vi "故障告警分析.vi"(8 "告警代码":u16, 9 "故障代码":u16, 10 "运行步序":u16, 11 "参数":string) -> (2 "报警内容":T1, 3 "简易报警状态":cluster{"故障状态":string, "报警状态":string})   [LabVIEW 2016, in "斯坦道总氮.lvlib"]
panel:
  # "1、注射泵水样阀口堵塞；\n2、注射泵阀过载或丝杆无动作。"
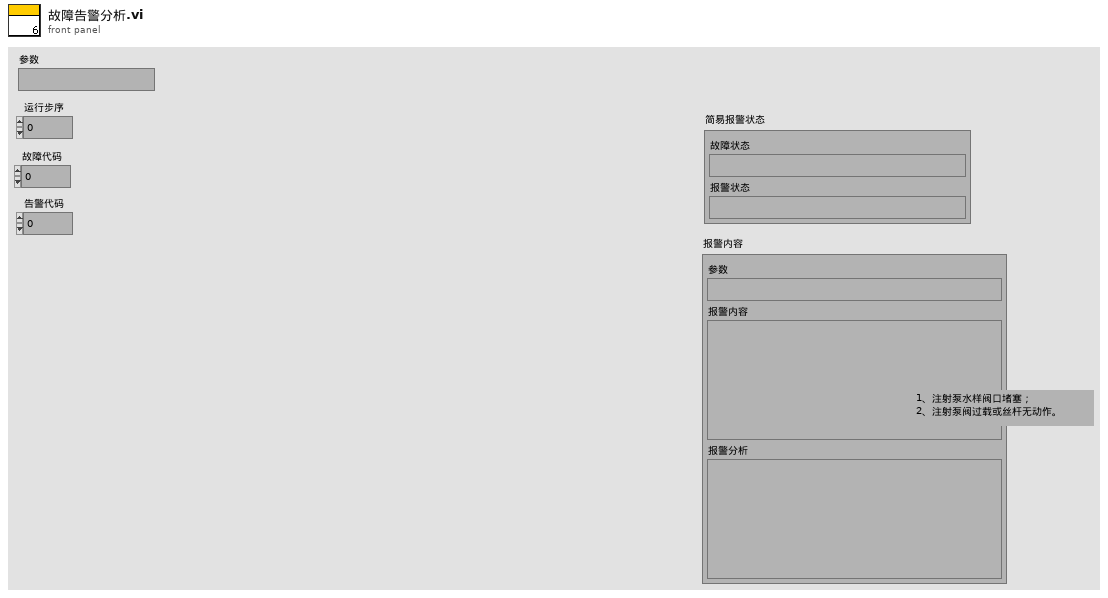
[diagram p1: front panel]
types:
  T1 = cluster{"参数":string, "报警内容":string, "报警分析":string}
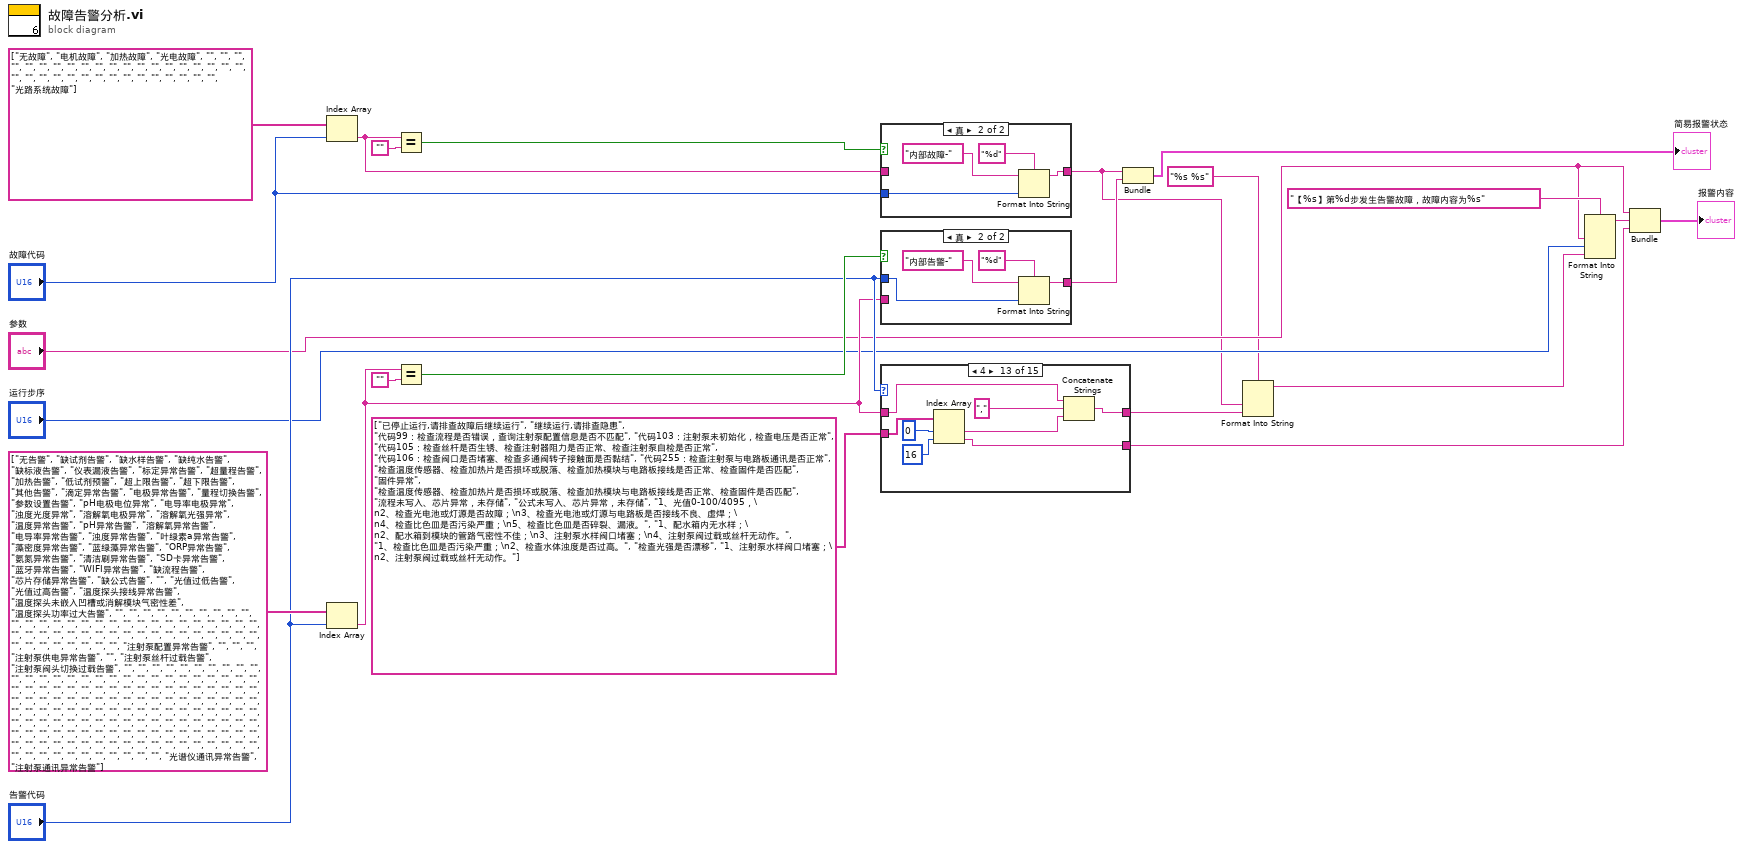
[diagram p0: block diagram]
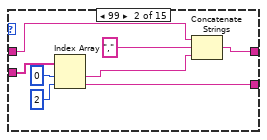
[diagram p3: hidden frame]
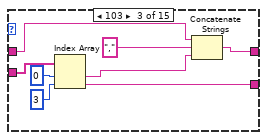
[diagram p4: hidden frame]
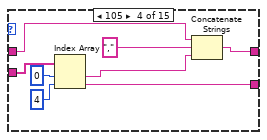
[diagram p5: hidden frame]
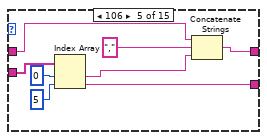
[diagram p6: hidden frame]
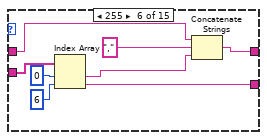
[diagram p7: hidden frame]
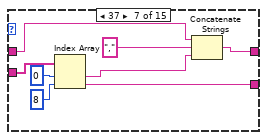
[diagram p8: hidden frame]
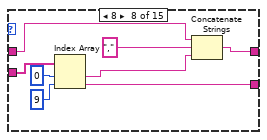
[diagram p9: hidden frame]
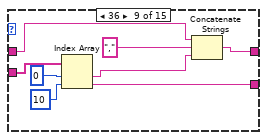
[diagram p10: hidden frame]
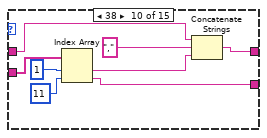
[diagram p11: hidden frame]
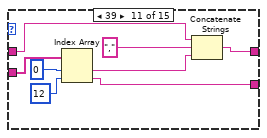
[diagram p12: hidden frame]
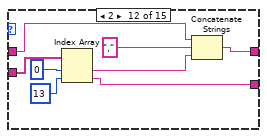
[diagram p13: hidden frame]
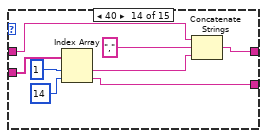
[diagram p14: hidden frame]
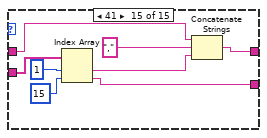
[diagram p15: hidden frame]
diagram:
  n1 = Index Array(array=string[] ["无故障", "电机故障", "加热故障", "光电故障", "", "", "", "", "", "", "", "", "", "", "", "", "", "", "", "", "", "", "", "", "", "", "", "", "", "", "", "", "", "", "", "", "", "", "", "光路系统故障"], index="故障代码") -> (element=w20:string)
  n2 = Index Array(array=string[] ["无告警", "缺试剂告警", "缺水样告警", "缺纯水告警", "缺标液告警", "仪表漏液告警", "标定异常告警", "超量程告警", "加热告警", "低试剂预警", "超上限告警", "超下限告警", "其他告警", "滴定异常告警", "电极异常告警", "量程切换告警", "参数设置告警", "pH电极电位异常", "电导率电极异常", "浊度光度异常", "溶解氧电极异常", "溶解氧光强异常", "温度异常告警", "pH异常告警", "溶解氧异常告警", "电导率异常告警", "浊度异常告警", "叶绿素a异常告警", "藻密度异常告警", "蓝绿藻异常告警", "ORP异常告警", "氨氮异常告警", "清洁刷异常告警", "SD卡异常告警", "蓝牙异常告警", "WIFI异常告警", "缺流程告警", "芯片存储异常告警", "缺公式告警", "", "光值过低告警", "光值过高告警", "温度探头接线异常告警", "温度探头未嵌入凹槽或消解模块气密性差", "温度探头功率过大告警", "", "", "", "", "", "", "", "", "", "", "", "", "", "", "", "", "", "", "", "", "", "", "", "", "", "", "", "", "", "", "", "", "", "", "", "", "", "", "", "", "", "", "", "", "", "", "", "", "", "", "", "", "", "", "注射泵配置异常告警", "", "", "", "注射泵供电异常告警", "", "注射泵丝杆过载告警", "注射泵阀头切换过载告警", "", "", "", "", "", "", "", "", "", "", "", "", "", "", "", "", "", "", "", "", "", "", "", "", "", "", "", "", "", "", "", "", "", "", "", "", "", "", "", "", "", "", "", "", "", "", "", "", "", "", "", "", "", "", "", "", "", "", "", "", "", "", "", "", "", "", "", "", "", "", "", "", "", "", "", "", "", "", "", "", "", "", "", "", "", "", "", "", "", "", "", "", "", "", "", "", "", "", "", "", "", "", "", "", "", "", "", "", "", "", "", "", "", "", "", "", "", "", "", "", "", "", "", "", "", "", "", "", "", "", "", "", "", "", "", "", "", "", "", "", "", "", "", "", "", "", "", "光谱仪通讯异常告警", "注射泵通讯异常告警"], index="告警代码") -> (element=w13:string)
  n3 = Equal?(x=w20, y="") -> (x = y?=w21:bool)
  n4 = Equal?(x=w13, y="") -> (x = y?=w16:bool)
  n5 = case shown="真" w21 {
    tunnel: [w24 w26] -> w2
    tunnel: w20 -> [w24 _]
    tunnel: "故障代码" -> [_ w25]
    frame False {
    }
    frame True {
      n6 = Format Into String(format string="%d" ("格式字符串"), initial string="内部故障-" ("工作状态"), w25) -> (resulting string=w26:string)  [unwired: 1 in, 1 out]
    }
  }
  n7 = case shown="真" w16 {
    tunnel: [w29 w31] -> w12
    tunnel: w13 -> [w29 _]
    tunnel: "告警代码" -> [_ w30]
    frame False {
    }
    frame True {
      n8 = Format Into String(format string="%d" ("格式字符串"), initial string="内部告警-" ("工作状态"), w30) -> (resulting string=w31:string)  [unwired: 1 in, 1 out]
    }
  }
  n9 = case shown="4" "告警代码" {
    tunnel: string[] ["已停止运行,请排查故障后继续运行", "继续运行,请排查隐患", "代码99：检查流程是否错误，查询注射泵配置信息是否不匹配", "代码103：注射泵未初始化，检查电压是否正常", "代码105：检查丝杆是否生锈、检查注射器阻力是否正常、检查注射泵自检是否正常", "代码106：检查阀口是否堵塞、检查多通阀转子接触面是否黏结", "代码255：检查注射泵与电路板通讯是否正常", "检查温度传感器、检查加热片是否损坏或脱落、检查加热模块与电路板接线是否正常、检查固件是否匹配", "固件异常", "检查温度传感器、检查加热片是否损坏或脱落、检查加热模块与电路板接线是否正常、检查固件是否匹配", "流程未写入、芯片异常，未存储", "公式未写入、芯片异常，未存储", "1、光值0-100/4095，\n2、检查光电池或灯源是否故障；\n3、检查光电池或灯源与电路板是否接线不良、虚焊；\n4、检查比色皿是否污染严重；\n5、检查比色皿是否碎裂、漏液。", "1、配水箱内无水样；\n2、配水箱到模块的管路气密性不佳；\n3、注射泵水样阀口堵塞；\n4、注射泵阀过载或丝杆无动作。", "1、检查比色皿是否污染严重；\n2、检查水体浊度是否过高。", "检查光强是否漂移", "1、注射泵水样阀口堵塞；\n2、注射泵阀过载或丝杆无动作。"] -> [_ w42 w50 w58 w66 w74 w82 w90 w98 w106 w114 w122 w130 w138 w146]
    tunnel: [w34 w37 w45 w53 w61 w69 w77 w85 w93 w101 w109 w117 w125 w133 w141] -> w3
    tunnel: [_ w38 w46 w54 w62 w70 w78 w86 w94 w102 w110 w118 w126 w134 w142] -> w10
    tunnel: w13 -> [w34 w36 w44 w52 w60 w68 w76 w84 w92 w100 w108 w116 w124 w132 w140]
    frame 0, Default {
    }
    frame 99 {
      n10 = Index Array(array=w42, index #1=0 ("索引"), index #2=2 ("索引")) -> (element #1=w40:string, element #2=w38:string)
      n11 = Concatenate Strings(w36, "," ("字符串"), w40) -> (w37:string)
    }
    frame 103 {
      n12 = Index Array(array=w50, index #1=0 ("索引"), index #2=3 ("索引")) -> (element #1=w48:string, element #2=w46:string)
      n13 = Concatenate Strings(w44, "," ("字符串"), w48) -> (w45:string)
    }
    frame 105 {
      n14 = Index Array(array=w58, index #1=0 ("索引"), index #2=4 ("索引")) -> (element #1=w56:string, element #2=w54:string)
      n15 = Concatenate Strings(w52, "," ("字符串"), w56) -> (w53:string)
    }
    frame 106 {
      n16 = Index Array(array=w66, index #1=0 ("索引"), index #2=5 ("索引")) -> (element #1=w64:string, element #2=w62:string)
      n17 = Concatenate Strings(w60, "," ("字符串"), w64) -> (w61:string)
    }
    frame 255 {
      n18 = Index Array(array=w74, index #1=0 ("索引"), index #2=6 ("索引")) -> (element #1=w72:string, element #2=w70:string)
      n19 = Concatenate Strings(w68, "," ("字符串"), w72) -> (w69:string)
    }
    frame 37 {
      n20 = Index Array(array=w82, index #1=0 ("索引"), index #2=8 ("索引")) -> (element #1=w80:string, element #2=w78:string)
      n21 = Concatenate Strings(w76, "," ("字符串"), w80) -> (w77:string)
    }
    frame 8 {
      n22 = Index Array(array=w90, index #1=0 ("索引"), index #2=9 ("索引")) -> (element #1=w88:string, element #2=w86:string)
      n23 = Concatenate Strings(w84, "," ("字符串"), w88) -> (w85:string)
    }
    frame 36 {
      n24 = Index Array(array=w98, index #1=0 ("索引"), index #2=10 ("索引")) -> (element #1=w96:string, element #2=w94:string)
      n25 = Concatenate Strings(w92, "," ("字符串"), w96) -> (w93:string)
    }
    frame 38 {
      n26 = Index Array(array=w106, index #1=1 ("索引"), index #2=11 ("索引")) -> (element #1=w104:string, element #2=w102:string)
      n27 = Concatenate Strings(w100, "," ("字符串"), w104) -> (w101:string)
    }
    frame 39 {
      n28 = Index Array(array=w114, index #1=0 ("索引"), index #2=12 ("索引")) -> (element #1=w112:string, element #2=w110:string)
      n29 = Concatenate Strings(w108, "," ("字符串"), w112) -> (w109:string)
    }
    frame 2 {
      n30 = Index Array(array=w122, index #1=0 ("索引"), index #2=13 ("索引")) -> (element #1=w120:string, element #2=w118:string)
      n31 = Concatenate Strings(w116, "," ("字符串"), w120) -> (w117:string)
    }
    frame 4 {
      n32 = Index Array(array=w130, index #1=0 ("索引"), index #2=16 ("索引")) -> (element #1=w128:string, element #2=w126:string)
      n33 = Concatenate Strings(w124, "," ("字符串"), w128) -> (w125:string)
    }
    frame 40 {
      n34 = Index Array(array=w138, index #1=1 ("索引"), index #2=14 ("索引")) -> (element #1=w136:string, element #2=w134:string)
      n35 = Concatenate Strings(w132, "," ("字符串"), w136) -> (w133:string)
    }
    frame 41 {
      n36 = Index Array(array=w146, index #1=1 ("索引"), index #2=15 ("索引")) -> (element #1=w144:string, element #2=w142:string)
      n37 = Concatenate Strings(w140, "," ("字符串"), w144) -> (w141:string)
    }
  }
  n38 = Bundle(w2, w12) -> (→"简易报警状态":cluster{string, string})  [unwired: 1 in]
  n39 = Format Into String(format string="%s %s" ("格式字符串"), w2, w3) -> (resulting string=w4:string)  [unwired: 2 in, 1 out]
  n40 = Format Into String(format string="【%s】第%d步发生告警故障，故障内容为%s" ("格式字符串"), "参数", "运行步序", w4) -> (resulting string=w8:string)  [unwired: 2 in, 1 out]
  n41 = Bundle("参数"="参数", w8, w10) -> (→"报警内容":cluster{"参数":string, string, string})  [unwired: 1 in]
